vi "Read Thermocouple Type.vi"(8 "error in (no error)":errorcluster, 11 "Thermocouple in":refnum<class "Thermocouple.lvclass">) -> (0 "error out":errorcluster, 2 "Thermocouple Type":T1, 3 "Thermocouple out":refnum<class "Thermocouple.lvclass">)   [LabVIEW 2018, in "Thermocouple.lvlib" / "Thermocouple.lvclass"]
uses:
  Thermocouple.lvclass
  Custom Controls/Thermocouple Type.ctl
  Thermocouple.lvclass/Thermocouple.ctl
  Thermocouple.lvlib
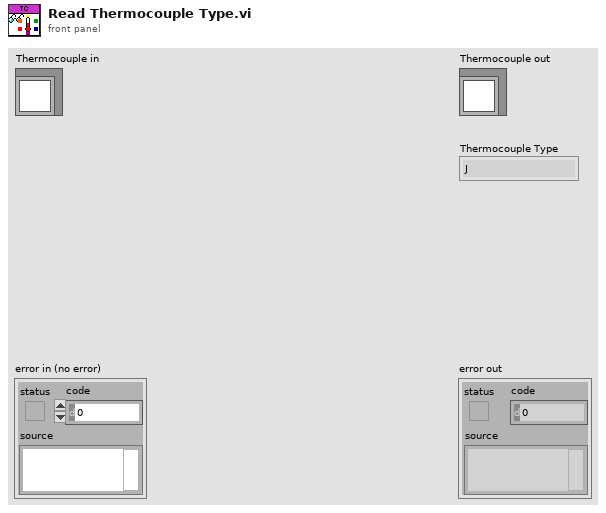
[diagram p1: front panel]
types:
  T1 = typedef "Thermocouple.lvlib/Thermocouple Type.ctl" = enum16{"J", "K", "N", "R", "S", "T", "B", "E"}
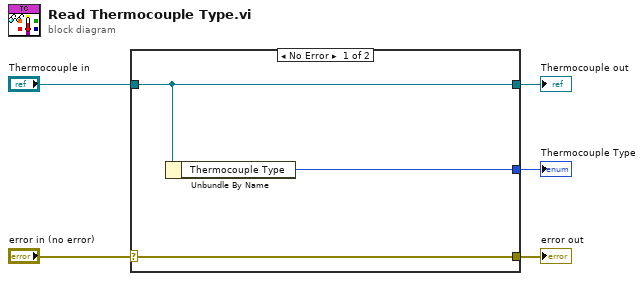
[diagram p0: block diagram]
diagram:
  n1 = case shown="No Error" "error in (no error)" {
    selector: "error in (no error)" -> [w8 w9]
    tunnel: [w8 w9] -> w4
    tunnel: [w7 w10] -> w2
    tunnel: "Thermocouple in" -> [w7 w10]
    tunnel: [w6 _] -> w1
    frame No Error {
      n2 = Unbundle By Name(w7) -> ("Thermocouple Type"=w6:T1)
    }
    frame Error {
    }
  }
  "error out" <- w4
  "Thermocouple out" <- w2
  "Thermocouple Type" <- w1
